vi "REPORT_REWORKS_get_data_from_SQL.vi"(7 "from_OP_to_OP":T1[](array[typedef]) items=["0"=0, "10"=10, "20"=20, "30"=30, "40"=40, "50"=50, "60"=60, "70"=70, "80"=80, "90"=90, "100"=100, "110"=110, "120"=120, "130"=130, "140"=140, "150"=150, "160"=160, "165"=165], 8 "error_in":errorcluster, 11 "dates_array":string[](array[string])) -> (0 "error_out":errorcluster, 3 "SQL_result":variant, 4 "executed_SQL_statement":string)   [LabVIEW 2019]
uses:
  typedef/REPORT_REWORKS_stations.ctl
  FGV/SQL_connection/FGV_CLIENT_SQL_connection.ctl
  FGV/REPORTS_records_display/FGV_REPORTS_records_display.ctl
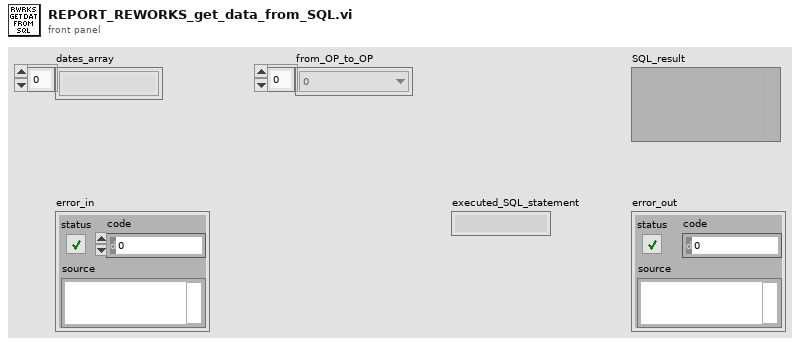
[diagram p1: front panel]
types:
  T1 = typedef "REPORT_REWORKS_stations.ctl" = u16
  T2 = typedef "FGV_REPORTS_records_display.ctl" = enum16{"initialize", "GEAR_set_serial", "GEAR_set_header", "GEAR_set_operations", "GEAR_set_results", "GEAR_set_batches", "GEAR_get_serial", "GEAR_get_operation_IDs", "GEAR_toggle_results", "GEAR_show_all_results", "GEAR_hide_all_results", "GEAR_display", "GEAR_filter", "GEAR_restore", "GEAR_clear", "GEAR_get_all_info", "DATES_set_dates", "DATES_set_gears", "DATES_display", "DATES_filter", "DATES_first_page", "DATES_previous_page", "DATES_next_page", "DATES_last_page", "DATES_restore", "DATES_clear", "DATES_get_all_info", "PBATCH_set_batch_no", "PBATCH_set_gears", "PBATCH_display", "PBATCH_filter", "PBATCH_first_page", "PBATCH_previous_page", "PBATCH_next_page", "PBATCH_last_page", "PBATCH_restore", "PBATCH_clear", "PBATCH_get_all_info", "OPRTN_set_OP", "OPRTN_set_dates", "OPRTN_set_gears", "OPRTN_set_hidden_columns", "OPRTN_display", "OPRTN_filter", "OPRTN_filter_no_page_reset", "OPRTN_first_page", "OPRTN_previous_page", "OPRTN_next_page", "OPRTN_last_page", "OPRTN_restore", "OPRTN_clear", "OPRTN_get_all_info", "CFG_set_type", "CFG_set_dates", "CFG_set_records", "CFG_display", "CFG_filter", "CFG_first_page", "CFG_previous_page", "CFG_next_page", "CFG_last_page", "CFG_restore", "CFG_clear", "CFG_get_all_info", "AUDIT_set_dates", "AUDIT_set_records", "AUDIT_display", "AUDIT_filter", "AUDIT_first_page", "AUDIT_previous_page", "AUDIT_next_page", "AUDIT_last_page", "AUDIT_restore", "AUDIT_clear", "AUDIT_get_all_info", "OKNOK_set_dates", "OKNOK_set_records", "OKNOK_display", "OKNOK_restore", "OKNOK_clear", "OKNOK_get_all_info", "REWORKS_set_dates", "REWORKS_set_from_to", "REWORKS_set_records", "REWORKS_display", "REWORKS_filter", "REWORKS_first_page", "REWORKS_previous_page", "REWORKS_next_page", "REWORKS_last_page", "REWORKS_restore", "REWORKS_clear", "REWORKS_get_all_info", "PACE_set_dates", "PACE_set_limits", "PACE_set_records", "PACE_display", "PACE_restore", "PACE_clear", "PACE_get_all_info", "CBATCH_set_code", "CBATCH_set_records", "CBATCH_display", "CBATCH_filter", "CBATCH_first_page", "CBATCH_previous_page", "CBATCH_next_page", "CBATCH_last_page", "CBATCH_restore", "CBATCH_clear", "CBATCH_get_all_info", "CMPNT_set_serial", "CMPNT_set_records", "CMPNT_display", "CMPNT_first_page", "CMPNT_previous_page", "CMPNT_next_page", "CMPNT_last_page", "CMPNT_restore", "CMPNT_clear", "CMPNT_get_all_info", "clear"}
  T3 = typedef "FGV_CLIENT_SQL_connection.ctl" = enum16{"initialize", "connect", "read_tables", "read_columns", "SELECT", "INSERT", "UPDATE", "DELETE", "EXEC + headers", "EXEC", "TRANSACTION", "connection_active?", "disconnect"}
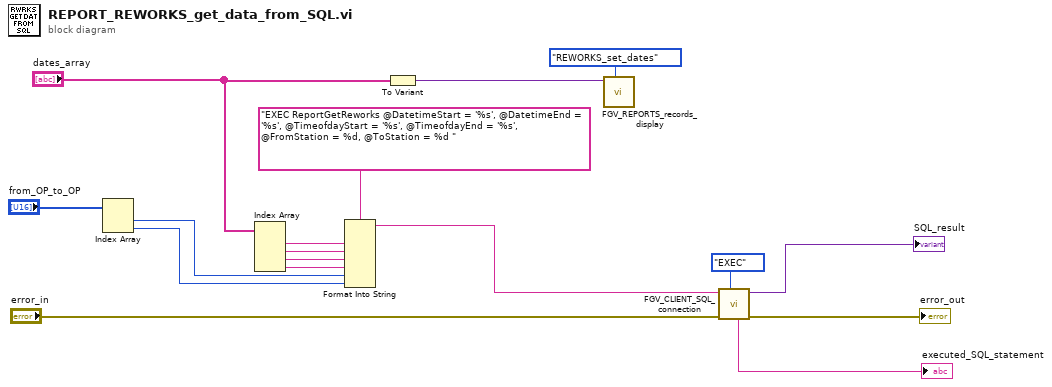
[diagram p0: block diagram]
diagram:
  n1 = Index Array(array="from_OP_to_OP") -> (element #1=w2:T1, element #2=w1:T1)  [unwired: 2 in]
  n2 = Index Array(array="dates_array") -> (element #1=w7:string, element #2=w6:string, element #3=w5:string, element #4=w4:string)  [unwired: 4 in]
  n3 = Format Into String(format string="EXEC ReportGetReworks @DatetimeStart = '%s', @DatetimeEnd = '%s', @TimeofdayStart = '%s', @TimeofdayEnd = '%s', @FromStation = %d, @ToStation = %d ", w7, w6, w5, w4, w2, w1) -> (resulting string=w13:string)  [unwired: 2 in, 1 out]
  n4 = To Variant(anything="dates_array") -> (Variant=w9:variant)
  n5 = call "FGV_REPORTS_records_display.vi"("options"=FGV_REPORTS_records_display."REWORKS_set_dates", "input"=w9) -> ()  [unwired: 8 in, 2 out]
  n6 = call "FGV_CLIENT_SQL_connection.vi"("options"=FGV_CLIENT_SQL_connection."EXEC", "error_in"="error_in", "SQL_statement"=w13) -> ("error_out"=→"error_out":errorcluster, "SQL_result"=→"SQL_result":variant, "executed_SQL_statement"=→"executed_SQL_statement":string)  [unwired: 4 in, 2 out]
